vi "TFTP Put File.vi"(5 "net address":string, 6 "Binary (T)":bool=TRUE, 7 "timeout ms (1000)":i32=1000, 8 "error in (no error)":errorcluster, 9 "local path":path, 10 "remote path":string, 11 "Host":string) -> (0 "error out":errorcluster, 2 "Status":bool, 3 "File Size":i64)   [LabVIEW 2013]
doc: "Connects to an TFTP server and copies the contents of a single file from the local machine."
panel:
  out "local port":u16
  out "file error":errorcluster
  out "server port":u16
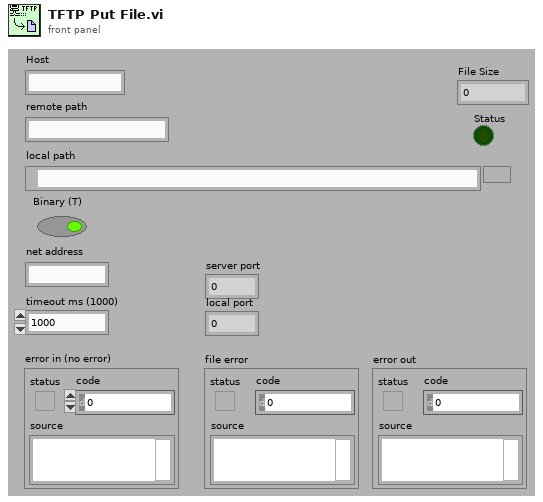
[diagram p1: front panel]
types:
  T1 = enum16{"open", "replace", "create", "open or create", "replace or create", "replace or create with confirmation"}
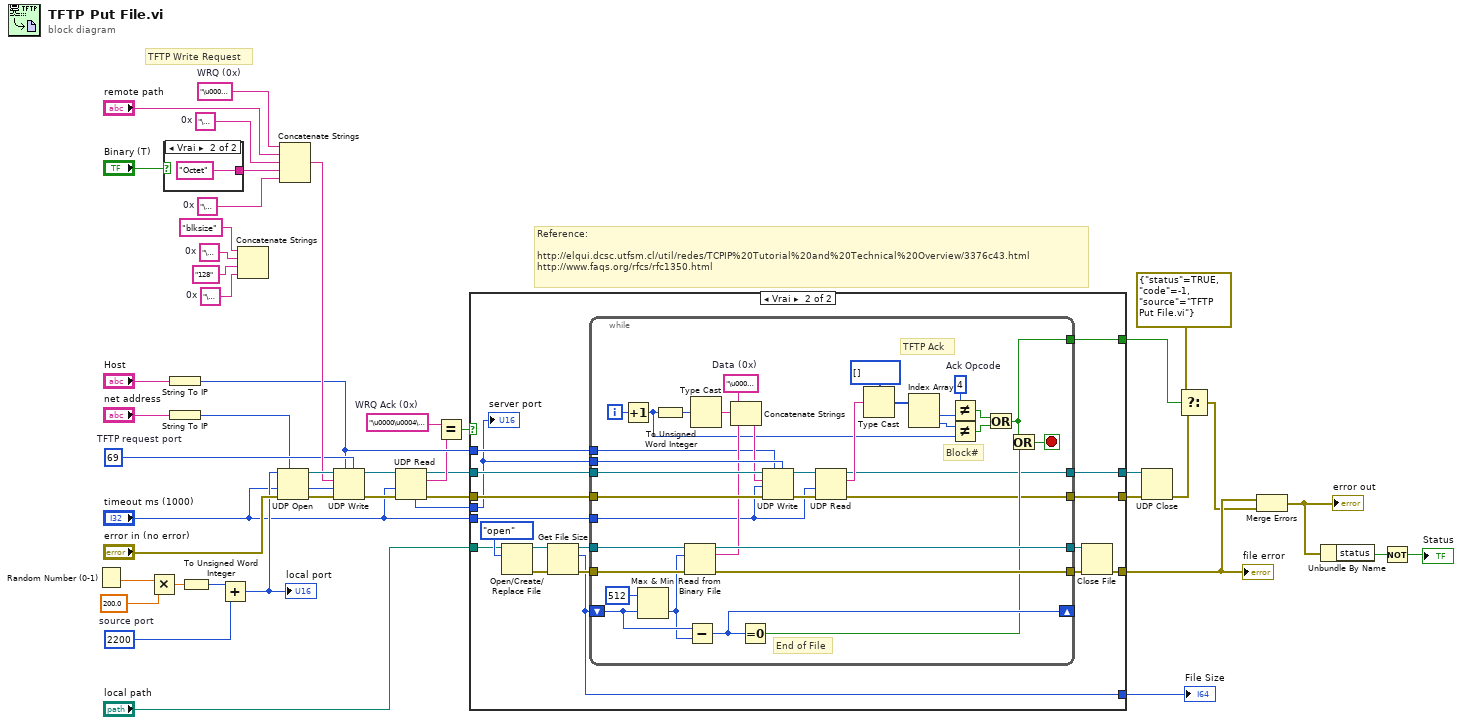
[diagram p0: block diagram]
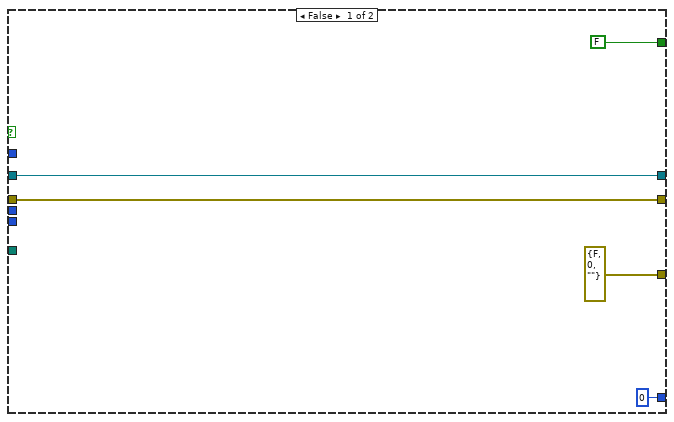
[diagram p2: hidden frame]
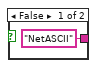
[diagram p3: hidden frame]
diagram:
  w1 = "\u0000"  # 0x
  w3 = "\u0000"  # 0x
  w21 = "\u0000\u0004\u0000\u0000"  # WRQ Ack (0x)
  w28 = u16 2200  # source port
  w38 = "\u0000"  # 0x
  w40 = "\u0000"  # 0x
  w42 = "\u0000\u0002"  # WRQ (0x)
  w34 = u16 69  # TFTP request port
  # "Reference:\n\nhttp://elqui.dcsc.utfsm.cl/util/redes/TCPIP%20Tutorial%20and%20Technical%20Overview/3376c43.html\nhttp://www.faqs.org/rfcs/rfc1350.html"
  # "TFTP Write Request"
  n1 = Random Number (0-1)() -> (number: 0 to 1=w30:dbl)
  n2 = Multiply(x=w30, y=200.0) -> (x*y=w32:dbl)
  n3 = case shown="Vrai" "Binary (T)" {
    tunnel: ["NetASCII" "Octet"] -> w39
    frame False {
    }
    frame True {
    }
  }
  n4 = String To IP(1:"Host") -> (0:w33:u32)
  n5 = String To IP(1:"net address") -> (0:w11:u32)
  n6 = To Unsigned Word Integer(number=w32) -> (unsigned 16bit integer=w29:u16)
  n7 = Add(x=w29, y=w28) -> (x+y=w27:u16)
  "local port" <- w27
  n8 = Concatenate Strings("blksize", w3, "128", w1) -> ()  [unwired: 1 out]
  n9 = UDP Open(7:w11, 8:"error in (no error)", 9:"timeout ms (1000)", 11:w27) -> (port=w45:refnum<k16>, 0:w44:errorcluster)  [unwired: 2 out]
  n10 = Concatenate Strings(w42, "remote path", w40, w39, w38) -> (w37:string)
  n11 = UDP Write(address=w33, port or service name=w34, connection ID=w45, data in=w37, 8:w44, 9:"timeout ms (1000)") -> (error out=w25:errorcluster, 3:w24:refnum<k16>)
  n12 = UDP Read(connection ID=w24, timeout ms (25000)="timeout ms (1000)", 8:w25) -> (data out=w22:string, error out=w18:errorcluster, 3:w19:refnum<k16>, 4:w17:u16)  [unwired: 2 out]
  n13 = Equal?(x=w21, y=w22) -> (x = y?=w20:bool)
  n14 = case shown="Vrai" w20 {
    tunnel: w33 -> [_ w71]
    tunnel: [FALSE w67] -> w14
    tunnel: [errorcluster {"status"=FALSE, "code"=0, "source"=""} ("error out") w66] -> w9
    tunnel: "local path" -> [_ w65]
    tunnel: "timeout ms (1000)" -> [_ w64]
    tunnel: w19 -> [w53 w63]
    tunnel: w18 -> [w52 w62]
    tunnel: w17 -> [_ w57]
    tunnel: [w52 w56] -> w16
    tunnel: [w53 w55] -> w15
    tunnel: [i64 0 ("size (in bytes)") w54] -> w10
    frame False {
    }
    frame True {
      n15 = Open/Create/Replace File(file path (use dialog)=w65, operation (0:open)=T1."open") -> (refnum out=w60:refnum<file>, error out=w61:errorcluster)  [unwired: 1 in, 4 out]
      n16 = Get File Size(file=w60, error in=w61) -> (refnum out=w58:refnum<file>, size (in bytes)=w54:i64, 0:w59:errorcluster)
      n17 = while {
        tunnel: w63 -> [w106]
        tunnel: w62 -> [w105]
        tunnel: w71 -> [w72]
        tunnel: w64 -> [w78]
        tunnel: [w95] -> w70
        tunnel: [w94] -> w69
        tunnel: [w93] -> w67
        tunnel: w57 -> [w92]
        shift-right: [w87] -> _
        shift-left: w54 -> [w89]
        tunnel: w59 -> [w90]
        tunnel: w58 -> [w86]
        tunnel: [w74] -> w56
        tunnel: [w73] -> w55
        i -> [w100]
        stop <- w97 stop-if-true
        w81 = "\u0000\u0003"  # Data (0x)
        w101 = u16 4  # Ack Opcode
        # "End of File"
        # "Block#"
        # "TFTP Ack"
        n18 = Increment(x=w100) -> (x+1=w76:i32)
        n19 = Max & Min(x=i64 512 ("count (1)"), y=w89) -> (min(x,y)=w88:i64)  [unwired: 1 out]
        n20 = To Unsigned Word Integer(number=w76) -> (unsigned 16bit integer=w83:u16)
        n21 = Read from Binary File(8:w90, 10:w88, 11:w86) -> (0:w94:errorcluster, 2:w79:string, 3:w95:refnum<file>)  [unwired: 4 out]
        n22 = Subtract(x=w89, y=w88) -> (x-y=w87:i64)
        n23 = Type Cast(x=w83) -> (*(type *) &x=w80:string)  [unwired: 1 out]
        n24 = Concatenate Strings(w81, w80, w79) -> (w82:string)
        n25 = Equal To 0?(x=w87) -> (x = 0?=w75:bool)
        n26 = UDP Write(address=w72, port or service name=w92, connection ID=w106, data in=w82, 8:w105, 9:w78) -> (error out=w84:errorcluster, 3:w85:refnum<k16>)
        n27 = UDP Read(connection ID=w85, timeout ms (25000)=w78, 8:w84) -> (data out=w77:string, error out=w74:errorcluster, 3:w73:refnum<k16>)  [unwired: 3 out]
        n28 = Type Cast(type=u16[] [], x=w77) -> (*(type *) &x=w103:u16[])
        n29 = Index Array(array=w103) -> (element #1=w102:u16, element #2=w96:u16)  [unwired: 2 in]
        n30 = Not Equal?(x=w101, y=w102) -> (x != y?=w98:bool)
        n31 = Not Equal?(x=w96, y=w76) -> (x != y?=w99:bool)
        n32 = Or(x=w98, y=w99) -> (x .or. y?=w93:bool)
        n33 = Or(x=w93, y=w75) -> (x .or. y?=w97:bool)
      }
      n34 = Close File(refnum=w70, error in=w69) -> (error out=w66:errorcluster)  [unwired: 1 out]
      "server port" <- w57
    }
  }
  "file error" <- w9
  "File Size" <- w10
  n35 = UDP Close(connection ID=w15, 8:w16) -> (error out=w13:errorcluster)  [unwired: 1 out]
  n36 = Select(t=errorcluster {"status"=TRUE, "code"=-1, "source"="TFTP Put File.vi"}, s=w14, f=w13) -> (s? t:f=w8:errorcluster)
  n37 = Merge Errors(w9, w8) -> (w7:errorcluster)
  "error out" <- w7
  n38 = Unbundle By Name(w7) -> ("status"=w6:bool)
  n39 = Not(x=w6) -> (.not. x?=→"Status":bool)
